vi "Parse Tag.vi"(11 "Tag String":string) -> (0 "</ Tag>":bool, 1 "Tag Name":string, 2 "Attributes":map{string, string}(c390))   [LabVIEW 2021, in "Tree Map.lvlib"]
doc: "<b>Author:</b> Piotr Kruczkowski <PrimaryKey>\n<b>License:</b> NewBSD\n\nCopyright (c) 2019, National Instruments\nAll rights reserved.\n\nRedistribution and use in source and binary forms, with or without\nmodification, are permitted provided that the following conditions are met:\n1. Redistributions of source code must retain the above copyright\n notice, this list of conditions and the following disclaimer.\n2. Redistributions in binary form must reproduce the above copyright\n notice, this list of conditions and the following disclaimer in the\n documentation and/or other materials provided with the distribution.\n3. Neither the name of National Instruments nor the\n names of its contributors may be used to endorse or promote products\n derived from this software without specific prior written permission.\n\nTHIS SOFTWARE IS PROVIDED BY National Instruments ''AS IS'' AND ANY\nEXPRESS OR IMPLIED WARRANTIES, INCLUDING, BUT NOT LIMITED TO, THE IMPLIED\nWARRANTIES OF MERCHANTABILITY AND FITNESS FOR A PARTICULAR PURPOSE ARE\nDISCLAIMED. IN NO EVENT SHALL National Instruments BE LIABLE FOR ANY\nDIRECT, INDIRECT, INCIDENTAL, SPECIAL, EXEMPLARY, OR CONSEQUENTIAL DAMAGES\n(INCLUDING, BUT NOT LIMITED TO, PROCUREMENT OF SUBSTITUTE GOODS OR SERVICES;\nLOSS OF USE, DATA, OR PROFITS; OR BUSINESS INTERRUPTION) HOWEVER CAUSED AND\nON ANY THEORY OF LIABILITY, WHETHER IN CONTRACT, STRICT LIABILITY, OR TORT\n(INCLUDING NEGLIGENCE OR OTHERWISE) ARISING IN ANY WAY OUT OF THE USE OF THIS\nSOFTWARE, EVEN IF ADVISED OF THE POSSIBILITY OF SUCH DAMAGE."
uses:
  <vilib>/National Instruments/Tree Map/Tree Map.lvlib
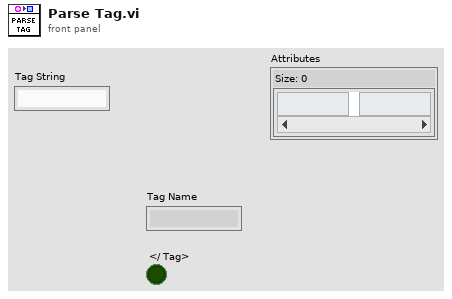
[diagram p1: front panel]
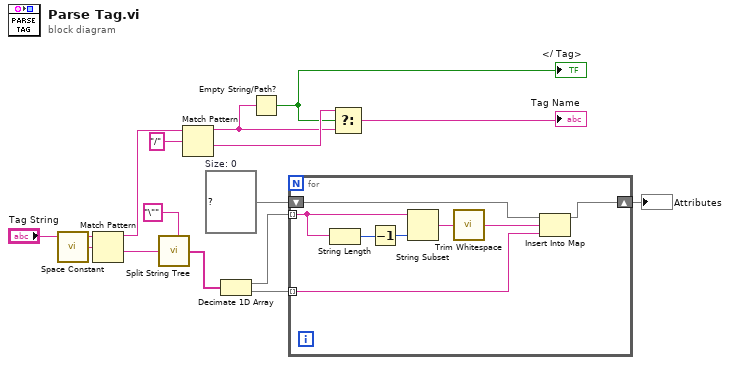
[diagram p0: block diagram]
diagram:
  w2 = map{string, string} {}  # Size: 0
  n1 = call <vilib>:"Space Constant.vi"() -> ("String"=w14:string)
  n2 = Match Pattern(string="Tag String", regular expression=w14) -> (before substring=w8:string, after substring=w13:string)  [unwired: 1 in, 2 out]
  n3 = call <vilib>:"Split String Tree.vi"("Split Pattern"="\"", "Input String"=w13) -> ("Split String"=w4:string[])  [unwired: 5 in]
  n4 = Match Pattern(string=w8, regular expression="/") -> (before substring=w9:string, after substring=w10:string)  [unwired: 1 in, 2 out]
  n5 = Decimate 1D Array(w4) -> (w5:string[], w3:string[])
  n6 = Empty String/Path?(string/path=w9) -> (empty?=w7:bool)
  "</ Tag>" <- w7
  n7 = for {
    tunnel: w5 -> [w22] mode=indexing
    tunnel: w3 -> [w18] mode=indexing
    shift-right: [w17] -> w1
    shift-left: w2 -> [w16]
    n8 = String Length(string=w22) -> (length=w21:i32)
    n9 = Decrement(x=w21) -> (x-1=w20:i32)
    n10 = String Subset(string=w22, length (rest)=w20) -> (substring=w23:string)  [unwired: 1 in]
    n11 = call <vilib>:"Trim Whitespace.vi"("string"=w23) -> ("trimmed string"=w19:string)  [unwired: 1 in]
    n12 = Insert Into Map(map in=w16, key=w19, value=w18) -> (map out=w17:map{string, string})  [unwired: 2 out]
  }
  "Attributes" <- w1
  n13 = Select(t=w10, s=w7, f=w9) -> (s? t:f=→"Tag Name":string)
